vi "Search Command Switch.vi"(10 "switches":cluster{"switch":string, "argument":string}[](array[cluster]), 11 "switch in":string) -> (1 "found?":bool, 2 "argument":string, 3 "switch out":string)   [LabVIEW 2017]
doc: "Searches for <b>switch in</b> in <b>switches</b>."
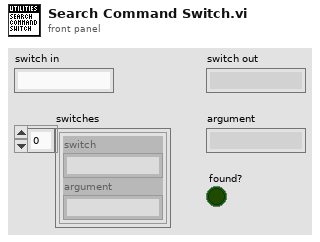
[diagram p1: front panel]
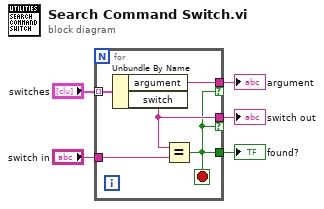
[diagram p0: block diagram]
diagram:
  n1 = for {
    tunnel: "switches" -> [w10] mode=indexing
    tunnel: "switch in" -> [w9]
    tunnel: [w6] -> w4
    tunnel: [w8] -> w2 if=w6
    tunnel: [w7] -> w1 if=w6
    stop <- w6 stop-if-true
    n2 = Unbundle By Name(w10) -> ("argument"=w8:string, "switch"=w7:string)
    n3 = Equal?(x=w7, y=w9) -> (x = y?=w6:bool)
  }
  "found?" <- w4
  "argument" <- w2
  "switch out" <- w1
